vi "Line follower.vi"   [LabVIEW 2015, in "ExemploFinal.lvrbt"]
uses:
  ExemploFinal.lvrbt
  <vilib>/NXT/Subs/MotorOutput.ctl
  <vilib>/NXT/Block Support/NXT_InputPort.ctl
  <vilib>/NXT/Block Support/NXT_ButtonSelector.ctl
  <vilib>/NXT/Dual Mode Library/Sensors/Light_On.vi
  <vilib>/NXT/Dual Mode Library/Sensors/readNXTButton.vi
  <vilib>/NXT/Dual Mode Library/Waits/Wait_Num(msec).vi
  <vilib>/NXT/Dual Mode Library/Motors/MotorOn.vi
  <vilib>/NXT/Dual Mode Library/Motors/MotorBrake.vi
panel:
  # "This code is designed to be deployed to the NXT brick. \nPress Ctrl + E  (Cmd + E on Mac) to show the block diagram and see the code."
types:
  T1 = typedef "MotorOutput.ctl" = u8
  T2 = typedef "NXT_InputPort.ctl" = u32
  T3 = typedef "NXT_ButtonSelector.ctl" = u16
  T4 = typedef "LVHSConnector.ctl" = refnum<class "BrickReference.lvclass">
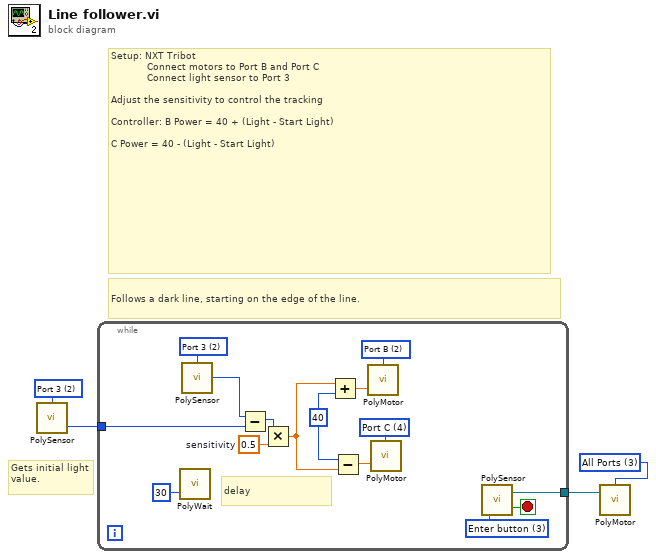
[diagram p0: block diagram]
diagram:
  w1 = T1 3 items=["Port A"=0, "Port B"=1, "Port C"=2, "Ports A & B"=4, "Ports A & C"=5, "Ports B & C"=6, "All Ports"=3] ("Output Port (All Ports)")
  w2 = T2 2 items=["Port 1", "Port 2", "Port 3", "Port 4"] ("Input Port (Port 3)")
  # "Follows a dark line, starting on the edge of the line."
  # "Gets initial light value."
  # "Setup: NXT Tribot\n            Connect motors to Port B and Port C\n            Connect light sensor to Port 3\n\nAdjust the sensitivity to control the tracking\n\nController: B Power = 40 + (Light - Start Light)\n\nC Power = 40 - (Light - Start Light)"
  n1 = call-poly <vilib>:"PolySensor.vi"("Port (Port 3)"=w2) -> ("Scaled Value"=w3:i16)  [unwired: 1 in, 2 out]
  n2 = while {
    tunnel: w3 -> [w14]
    tunnel: [w5] -> w4
    stop <- w13 stop-if-true
    w6 = 0.5  # sensitivity
    w9 = T1 4 items=["Port A"=1, "Port B"=2, "Port C"=4, "A & B"=3, "A & C"=5, "B & C"=6, "All Ports"=7] ("Output Port (All Ports)")
    w10 = T1 2 items=["Port A"=1, "Port B"=2, "Port C"=4, "A & B"=3, "A & C"=5, "B & C"=6, "All Ports"=7] ("Output Port (All Ports)")
    w12 = T3 3 items=["Enter button"=3, "Left button"=2, "Right button"=1] ("Button (Enter button)")
    w16 = 40 ("y")
    w19 = T2 2 items=["Port 1", "Port 2", "Port 3", "Port 4"] ("Input Port (Port 3)")
    # "delay"
    n3 = call-poly <vilib>:"PolyWait.vi"("Time (100 msec)"=u32 30 ("Time (1 sec)")) -> ()  [unwired: 3 in, 1 out]
    n4 = call-poly <vilib>:"PolySensor.vi"("Port (Port 3)"=w19) -> ("Scaled Value"=w18:i16)  [unwired: 1 in, 2 out]
    n5 = Subtract(x=w18, y=w14) -> (x-y=w8:i16)
    n6 = Multiply(x=w8, y=w6) -> (x*y=w7:dbl)
    n7 = Add(x=w7, y=w16) -> (x+y=w17:dbl)
    n8 = Subtract(x=w16, y=w7) -> (x-y=w15:dbl)
    n9 = call-poly <vilib>:"PolyMotor.vi"("Power (75)"=w17, "Output Port (All Ports)"=w10) -> ()  [unwired: 1 in, 2 out]
    n10 = call-poly <vilib>:"PolyMotor.vi"("Power (75)"=w15, "Output Port (All Ports)"=w9) -> ()  [unwired: 1 in, 2 out]
    n11 = call-poly <vilib>:"PolySensor.vi"("Button (Enter button)"=w12) -> ("Yes/No"=w13:bool, "NXT/EV3"=w5:T4)  [unwired: 1 in, 1 out]
  }
  n12 = call-poly <vilib>:"PolyMotor.vi"("NXT/EV3"=w4, "Port (All Ports)"=w1) -> ()  [unwired: 3 out]
